vi "PV Getting Started.vi"(0 "COM Port Name in":string="COM1", 1 "Adress of unit":u16=1 min=1 max=999 step=1, 5 "error in (no error)":errorcluster) -> (12 "Unit adress":string, 14 "Set rotation speed TMP [Hz]":string, 15 "Operating hours TMP [h]":string, 16 "Unit type electronic drive unit":string, 17 "Software version electronic drive unit":string, 18 "Operating hours electronic drive unit [h]":string, 19 "error out":errorcluster {"code" format="%.0x"})   [LabVIEW 2016, in "Pfeiffer Vacuum.lvlib"]
doc: "This VI is an example of how to use the Pfeiffer Vacuum subVIs programmatically. This VI first initializes the instrument, takes measurements, then closes the instrument.\n\nWARNINGS: \nYou MUSThave VISA Version 2.0 or higher installed to use this Instrument driver."
uses:
  Pfeiffer Vacuum.lvlib
  PV Miscellaneous - Cluster.ctl
  PV Operating adjustment - Cluster.ctl
panel:
  # "pump"
  # "electronic drive unit"
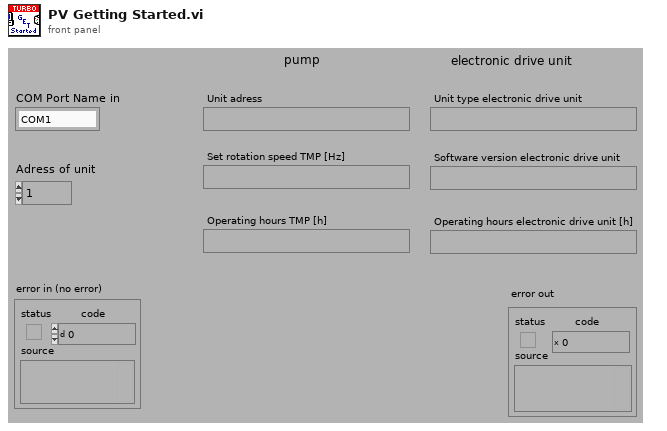
[diagram p1: front panel]
types:
  T1 = typedef "Pfeiffer Vacuum.lvlib/PV Operating adjustment - Cluster.ctl" = cluster{"Parameter":u16, "Parameter\nread only<->describe":bool, "off<->on":bool, "Rotation speed set value\nin rot. speed setting\noperations [%]":dbl, "Preset rotation Speed\nat Standby mode (%)":dbl, "maximum power\nsetpoint [%]":i32, "Gas mode":u16}
  T2 = typedef "Pfeiffer Vacuum.lvlib/PV Miscellaneous - Cluster.ctl" = cluster{"Parameter":u16, "Parameter\nread only<->describe":bool, "off<->on   ":bool, "Unit adress":i16, "Configuration AO1 (old version)":u16, "Contens of service\nline; # of the 2nd\n parameter":i16, "Configuration DO1 (old version)":u16}
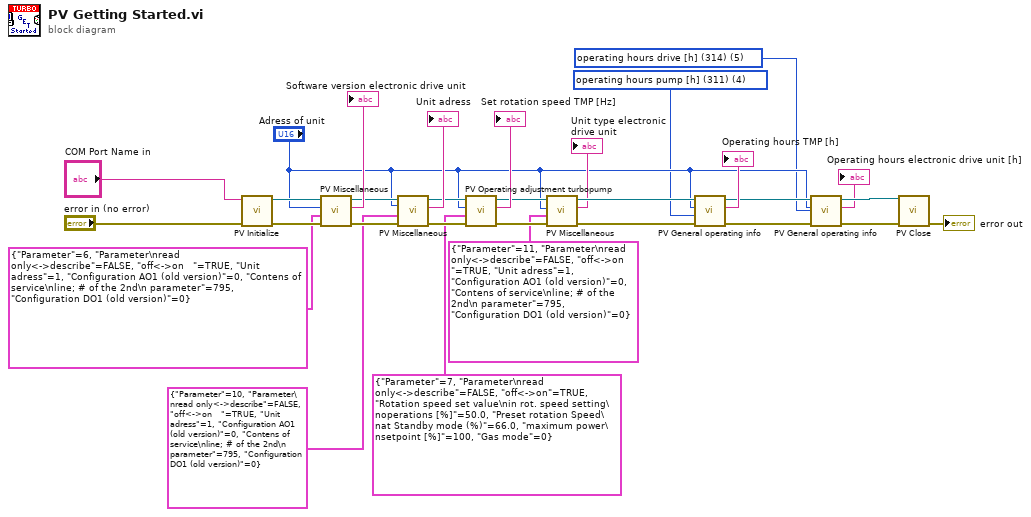
[diagram p0: block diagram]
diagram:
  w5 = u16 5 items=["nominal speed [Hz] (default) (315)", "intermediate circut current [A] (310)", "motor voltage [V] (313)", "actual power [W] (316)", "operating hours pump [h] (311)", "operating hours drive [h] (314)", "pump cycles (read only) (319)", "status oil sensor (read only) (301)", "speed switchpoint attained (read only) (302)", "overtemperature drive (read only) (304)", "overtemperature pump (read only) (305)", "target speed attained (read only) (306)", "pump accelerates (read only) (307) "] ("Parameter")
  w6 = u16 4 items=["nominal speed [Hz] (default) (315)", "intermediate circut current [A] (310)", "motor voltage [V] (313)", "actual power [W] (316)", "operating hours pump [h] (311)", "operating hours drive [h] (314)", "pump cycles (read only) (319)", "status oil sensor (read only) (301)", "speed switchpoint attained (read only) (302)", "overtemperature drive (read only) (304)", "overtemperature pump (read only) (305)", "target speed attained (read only) (306)", "pump accelerates (read only) (307) "] ("Parameter")
  n1 = call "PV Initialize.vi"("error in (no error)"="error in (no error)", "VISA session in"="COM Port Name in") -> ("error out"=w27:errorcluster, "VISA session out"=w28:refnum<visa-resource-name>)  [unwired: 8 in]
  n2 = call "PV Miscellaneous.vi"("error in (no error)"=w27, "PV Miscellaneous - Cluster"=T2 {"Parameter"=6, "Parameter\nread only<->describe"=FALSE, "off<->on   "=TRUE, "Unit adress"=1, "Configuration AO1 (old version)"=0, "Contens of service\nline; # of the 2nd\n parameter"=795, "Configuration DO1 (old version)"=0}, "Adress of unit"="Adress of unit", "VISA session"=w28) -> ("error out"=w24:errorcluster, "response (data)"=→"Software version electronic drive unit":string, "dup VISA session"=w25:refnum<visa-resource-name>)  [unwired: 5 in]
  n3 = call "PV Miscellaneous.vi"("error in (no error)"=w24, "PV Miscellaneous - Cluster"=T2 {"Parameter"=10, "Parameter\nread only<->describe"=FALSE, "off<->on   "=TRUE, "Unit adress"=1, "Configuration AO1 (old version)"=0, "Contens of service\nline; # of the 2nd\n parameter"=795, "Configuration DO1 (old version)"=0}, "Adress of unit"="Adress of unit", "VISA session"=w25) -> ("error out"=w21:errorcluster, "response (data)"=→"Unit adress":string, "dup VISA session"=w22:refnum<visa-resource-name>)  [unwired: 5 in]
  n4 = call "PV Operating adjustment turbopump.vi"("error in (no error)"=w21, "Operating adjustment - Cluster"=T1 {"Parameter"=7, "Parameter\nread only<->describe"=FALSE, "off<->on"=TRUE, "Rotation speed set value\nin rot. speed setting\noperations [%]"=50.0, "Preset rotation Speed\nat Standby mode (%)"=66.0, "maximum power\nsetpoint [%]"=100, "Gas mode"=0}, "Adress of unit"="Adress of unit", "VISA session"=w22) -> ("error out"=w12:errorcluster, "response (data)"=→"Set rotation speed TMP [Hz]":string, "dup VISA session"=w13:refnum<visa-resource-name>)  [unwired: 5 in]
  n5 = call "PV Miscellaneous.vi"("error in (no error)"=w12, "PV Miscellaneous - Cluster"=T2 {"Parameter"=11, "Parameter\nread only<->describe"=FALSE, "off<->on   "=TRUE, "Unit adress"=1, "Configuration AO1 (old version)"=0, "Contens of service\nline; # of the 2nd\n parameter"=795, "Configuration DO1 (old version)"=0}, "Adress of unit"="Adress of unit", "VISA session"=w13) -> ("error out"=w10:errorcluster, "response (data)"=→"Unit type electronic drive unit":string, "dup VISA session"=w11:refnum<visa-resource-name>)  [unwired: 5 in]
  n6 = call "PV General operating info.vi"("error in (no error)"=w10, "Parameter"=w6, "Adress of unit"="Adress of unit", "VISA session"=w11) -> ("error out"=w16:errorcluster, "response (data)"=→"Operating hours TMP [h]":string, "dup VISA session"=w18:refnum<visa-resource-name>)  [unwired: 5 in]
  n7 = call "PV General operating info.vi"("error in (no error)"=w16, "Parameter"=w5, "Adress of unit"="Adress of unit", "VISA session"=w18) -> ("error out"=w15:errorcluster, "response (data)"=→"Operating hours electronic drive unit [h]":string, "dup VISA session"=w17:refnum<visa-resource-name>)  [unwired: 5 in]
  n8 = call "PV Close.vi"("VISA session"=w17, "error in (no error)"=w15) -> ("error out"=→"error out":errorcluster)  [unwired: 13 in]
